vi "Shift_007.vi"() -> ()   [LabVIEW 2019]
panel:
  out "Force Chart":cluster{dbl[unit], dbl[unit]}(graph)
  out "Energies":dbl[unit][][](array[numeric])
  out "Energies":dbl[unit][][](graph)
  in  "time threshold 2":dbl[unit]=5.0
  in  "Control Force 2":dbl[unit]=1000.0
  in  "time threshold 1":dbl[unit]=2.0
  in  "Control Force 1":dbl[unit]=1000.0
  in  "D":dbl[unit]=25.0
  out "Ep(tk)":dbl[unit][](array[numeric])
  out "Et(tk)":dbl[unit][](array[numeric])
  out "Ek(tk)":dbl[unit][](array[numeric])
  out "Et":cluster{dbl[unit][], dbl[unit][]}(graph)
  out "Ep":cluster{dbl[unit][], dbl[unit][]}(graph)
  out "Ek":cluster{dbl[unit][], dbl[unit][]}(graph)
  out "Et":dbl[unit][](graph)
  out "Ep":dbl[unit][](graph)
  out "Ek":dbl[unit][](graph)
  out "a":cluster{dbl[unit][], dbl[unit][]}(graph)
  out "v":cluster{dbl[unit][], dbl[unit][]}(graph)
  out "x":cluster{dbl[unit][], dbl[unit][]}(graph)
  out "time (tk)":dbl[unit][](array[numeric])
  out "a":dbl[unit][](graph)
  out "v":dbl[unit][](graph)
  out "x":dbl[unit][](graph)
  out "x(tk)":dbl[unit][](array[numeric])
  out "v(tk)":dbl[unit][](array[numeric])
  out "a(tk)":dbl[unit][](array[numeric])
  in  "M":dbl[unit]=100.0
  in  "k":dbl[unit]=1000.0
  in  "v0":dbl[unit]
  in  "x0":dbl[unit]=2.0
  in  "Dt":dbl[unit]=1e-05
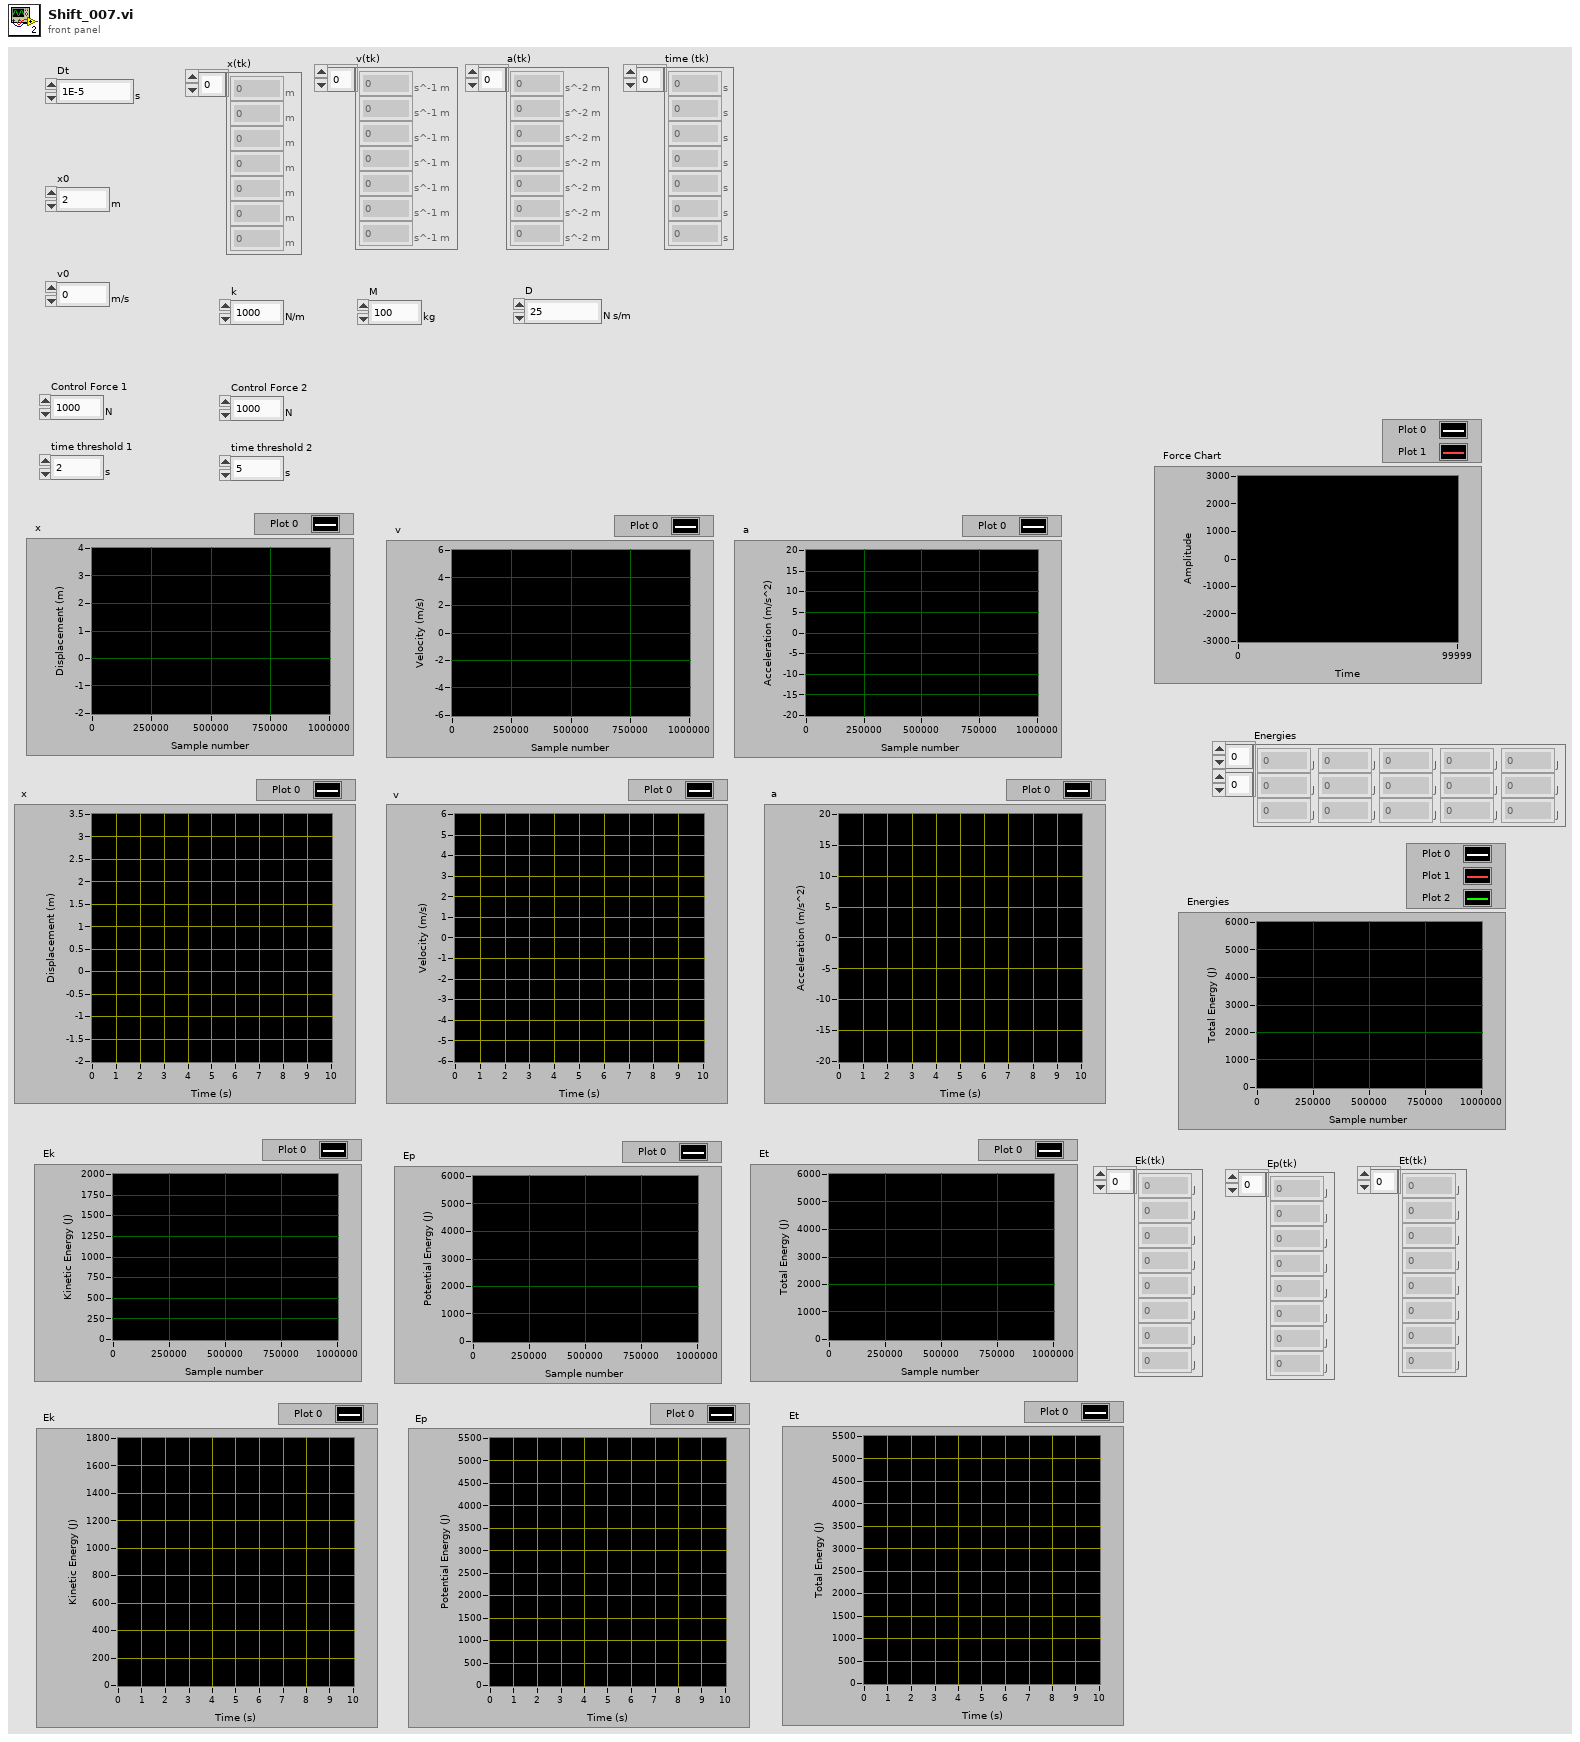
[diagram p1: front panel]
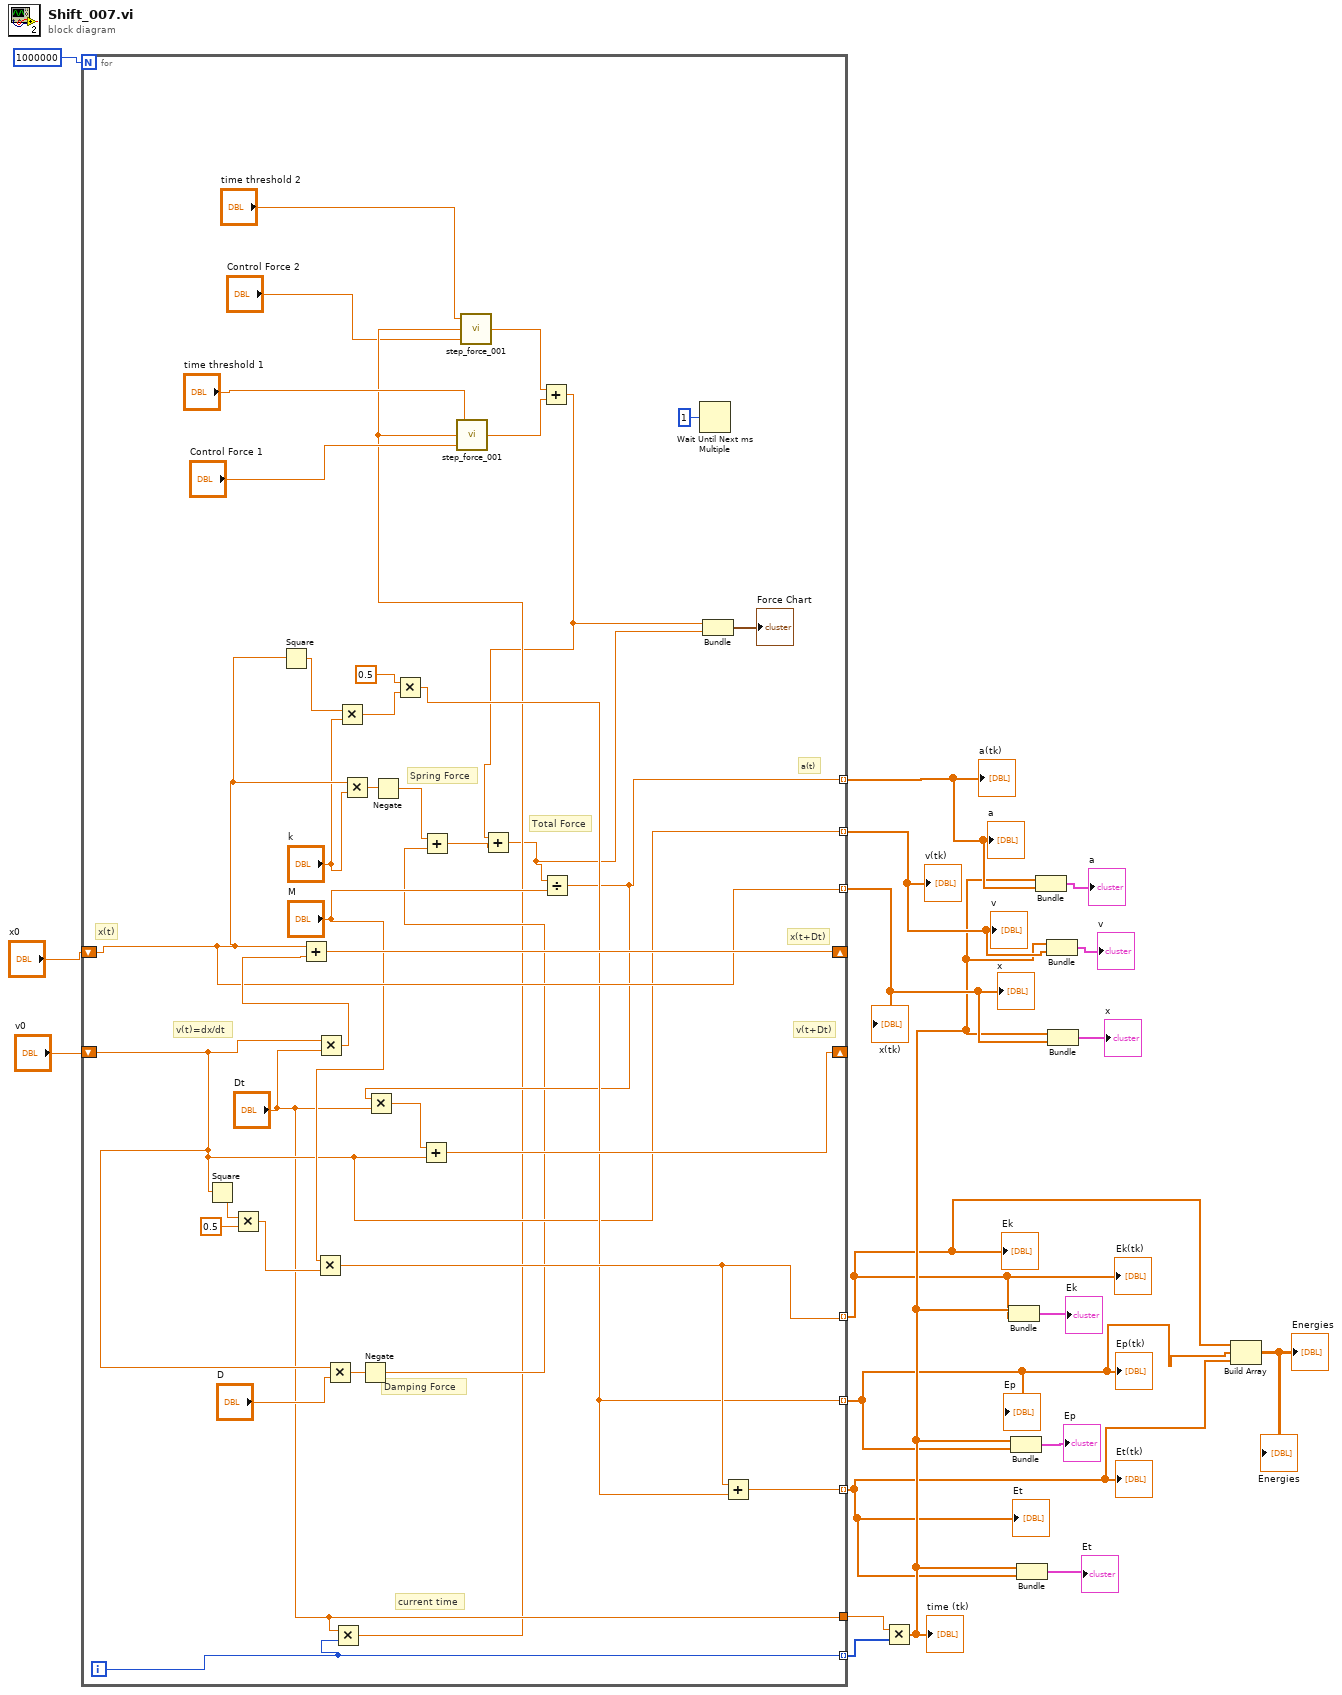
[diagram p0: block diagram]
diagram:
  n1 = for {
    N: 1000000 -> [_]
    shift-right: [w55] -> _
    shift-left: "x0" -> [w49]
    shift-right: [w52] -> _
    shift-left: "v0" -> [w39]
    tunnel: [w35] -> w11 mode=indexing
    tunnel: [w39] -> w10 mode=indexing
    tunnel: [w49] -> w9 mode=indexing
    tunnel: [w31] -> w15 mode=indexing
    tunnel: ["Dt"] -> w16
    tunnel: [w44] -> w4 mode=indexing
    tunnel: [w41] -> w3 mode=indexing
    tunnel: [w43] -> w2 mode=indexing
    i -> [w31]
    # "Total Force"
    # "current time"
    # "Spring Force"
    # "Damping Force"
    # "a(t)"
    # "v(t+Dt)"
    # "x(t+Dt)"
    # "v(t)=dx/dt"
    # "x(t)"
    n2 = Square(x=w39) -> (x^2=w50:dbl[unit])
    n3 = Multiply(x=w50, y=0.5) -> (x*y=w45:dbl[unit])
    n4 = Square(x=w49) -> (x^2=w48:dbl[unit])
    n5 = Multiply(x="M", y=w45) -> (x*y=w44:dbl[unit])
    n6 = Multiply(x=w39, y="Dt") -> (x*y=w56:dbl[unit])
    n7 = Add(x=w49, y=w56) -> (x+y=w55:dbl[unit])
    n8 = Multiply(x=w39, y="D") -> (x*y=w38:dbl[unit])
    n9 = Multiply(x="Dt", y=w31) -> (x*y=w28:dbl[unit])
    n10 = Multiply(x=w48, y="k") -> (x*y=w47:dbl[unit])
    n11 = Multiply(x=w49, y="k") -> (x*y=w54:dbl[unit])
    n12 = Negate(x=w38) -> (-x=w34:dbl[unit])
    n13 = Negate(x=w54) -> (-x=w36:dbl[unit])
    n14 = Multiply(x=0.5, y=w47) -> (x*y=w41:dbl[unit])
    n15 = Add(x=w36, y=w34) -> (x+y=w33:dbl[unit])
    n16 = call "step_force_001.vi"("Control Force in"="Control Force 1", "Current time"=w28, "time threshold"="time threshold 1") -> ("Control Force out"=w25:dbl[unit])
    n17 = call "step_force_001.vi"("Control Force in"="Control Force 2", "Current time"=w28, "time threshold"="time threshold 2") -> ("Control Force out"=w24:dbl[unit])
    n18 = Add(x=w24, y=w25) -> (x+y=w23:dbl[unit])
    n19 = Add(x=w23, y=w33) -> (x+y=w22:dbl[unit])
    n20 = Divide(x=w22, y="M") -> (x/y=w35:dbl[unit])
    n21 = Multiply(x=w35, y="Dt") -> (x*y=w53:dbl[unit])
    n22 = Add(x=w53, y=w39) -> (x+y=w52:dbl[unit])
    n23 = Wait Until Next ms Multiple(millisecond multiple=u32 1) -> ()  [unwired: 1 out]
    n24 = Bundle(w23, w22) -> (→"Force Chart":cluster{dbl[unit], dbl[unit]})  [unwired: 1 in]
    n25 = Add(x=w44, y=w41) -> (x+y=w43:dbl[unit])
  }
  "a(tk)" <- w11
  "v(tk)" <- w10
  "x(tk)" <- w9
  "v" <- w10
  "a" <- w11
  "x" <- w9
  "Et" <- w2
  "Ek" <- w4
  "Ep" <- w3
  "Ek(tk)" <- w4
  "Et(tk)" <- w2
  "Ep(tk)" <- w3
  n26 = Multiply(x=w16, y=w15) -> (x*y=w5:dbl[unit][])
  "time (tk)" <- w5
  n27 = Bundle(w5, w4) -> (→"Ek":cluster{dbl[unit][], dbl[unit][]})  [unwired: 1 in]
  n28 = Bundle(w5, w3) -> (→"Ep":cluster{dbl[unit][], dbl[unit][]})  [unwired: 1 in]
  n29 = Bundle(w5, w2) -> (→"Et":cluster{dbl[unit][], dbl[unit][]})  [unwired: 1 in]
  n30 = Bundle(w5, w11) -> (→"a":cluster{dbl[unit][], dbl[unit][]})  [unwired: 1 in]
  n31 = Bundle(w5, w10) -> (→"v":cluster{dbl[unit][], dbl[unit][]})  [unwired: 1 in]
  n32 = Bundle(w5, w9) -> (→"x":cluster{dbl[unit][], dbl[unit][]})  [unwired: 1 in]
  n33 = Build Array(w4, w3, w2) -> (→"Energies" →"Energies":dbl[unit][][])
